vi "GetAssetsDirectory.vi"(8 "error in":errorcluster, 11 "test VI refnum":refnum<vi>) -> (0 "error out":errorcluster, 3 "assets dir":path)   [LabVIEW 2027, in "VeriStandTestUtilities.lvlib"]
uses:
  VeriStandTestUtilities.lvlib
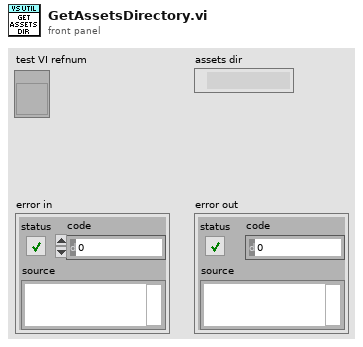
[diagram p1: front panel]
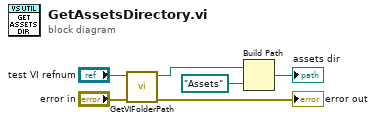
[diagram p0: block diagram]
diagram:
  n1 = call "GetVIFolderPath.vi"("error in (no error)"="error in", "VI Reference in"="test VI refnum") -> ("error out"=→"error out":errorcluster, "VI Folder Path out"=w6:path)  [unwired: 8 in]
  n2 = Build Path(base path=w6, name or relative path=path "Assets") -> (appended path=→"assets dir":path)
